vi "Name Label Opposite Visible Read.vi"(8 "error in (no error)":errorcluster, 11 "3D Plot.lvclass in":refnum<class "3D Plot.lvclass">) -> (0 "error out":errorcluster, 1 "Caption Opposite Visible?":bool, 3 "3D Plot.lvclass out":refnum<class "3D Plot.lvclass">)   [LabVIEW 2017, in "3D Plot.lvclass"]
uses:
  <vilib>/Math Plots/3D Math Plots/3D Plot/3D Plot/3D Plot.lvclass
  <vilib>/Math Plots/3D Math Plots/3D Plot/3D Plot/3D Plot.lvclass/3D Plot.ctl
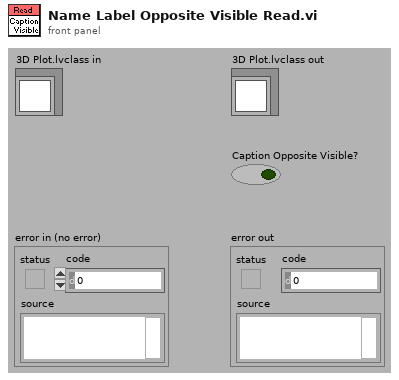
[diagram p1: front panel]
types:
  T1 = cluster{"Show Normal X Caption":bool, "Show Normal Y Caption":bool, "Show Normal Z Caption":bool, "Show Opposite X Caption":bool, "Show Opposite Y Caption":bool, "Show Opposite Z Caption":bool}
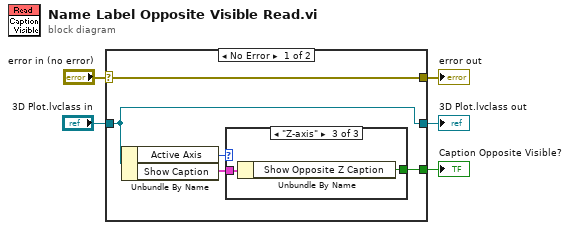
[diagram p0: block diagram]
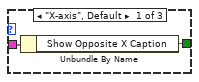
[diagram p2: hidden frame]
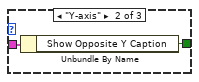
[diagram p3: hidden frame]
diagram:
  n1 = case shown="No Error" "error in (no error)" {
    selector: "error in (no error)" -> [w7 w17]
    tunnel: [w10 _] -> w5
    tunnel: "3D Plot.lvclass in" -> [w6 w18]
    tunnel: [w7 w17] -> w2
    tunnel: [w6 w18] -> w1
    frame No Error {
      n2 = Unbundle By Name(w6) -> ("Active Axis"=w8:enum16{"X-axis", "Y-axis", "Z-axis"}, "Show Caption"=w9:T1)
      n3 = case shown="\"Z-axis\"" w8 {
        tunnel: w9 -> [w11 w14 w16]
        tunnel: [w12 w13 w15] -> w10
        frame "X-axis", Default {
          n4 = Unbundle By Name(w11) -> ("Show Opposite X Caption"=w12:bool)
        }
        frame "Y-axis" {
          n5 = Unbundle By Name(w14) -> ("Show Opposite Y Caption"=w13:bool)
        }
        frame "Z-axis" {
          n6 = Unbundle By Name(w16) -> ("Show Opposite Z Caption"=w15:bool)
        }
      }
    }
    frame Error {
    }
  }
  "error out" <- w2
  "Caption Opposite Visible?" <- w5
  "3D Plot.lvclass out" <- w1
